vi "Path length, indv indice.vi"(11 "Raw position":dbl[][](array[numeric])) -> (3 "Path length data":dbl[][](array[numeric]))   [LabVIEW 2020]
panel:
  out "Path lenght data":dbl[](array[numeric])
  out "deleted portion":dbl[][](array[numeric])
  out "Path length upper shoulder":dbl
  out "path lenght Wrist":dbl
  out "path lenght elbow":dbl
  out "path lenght lower shoulder":dbl
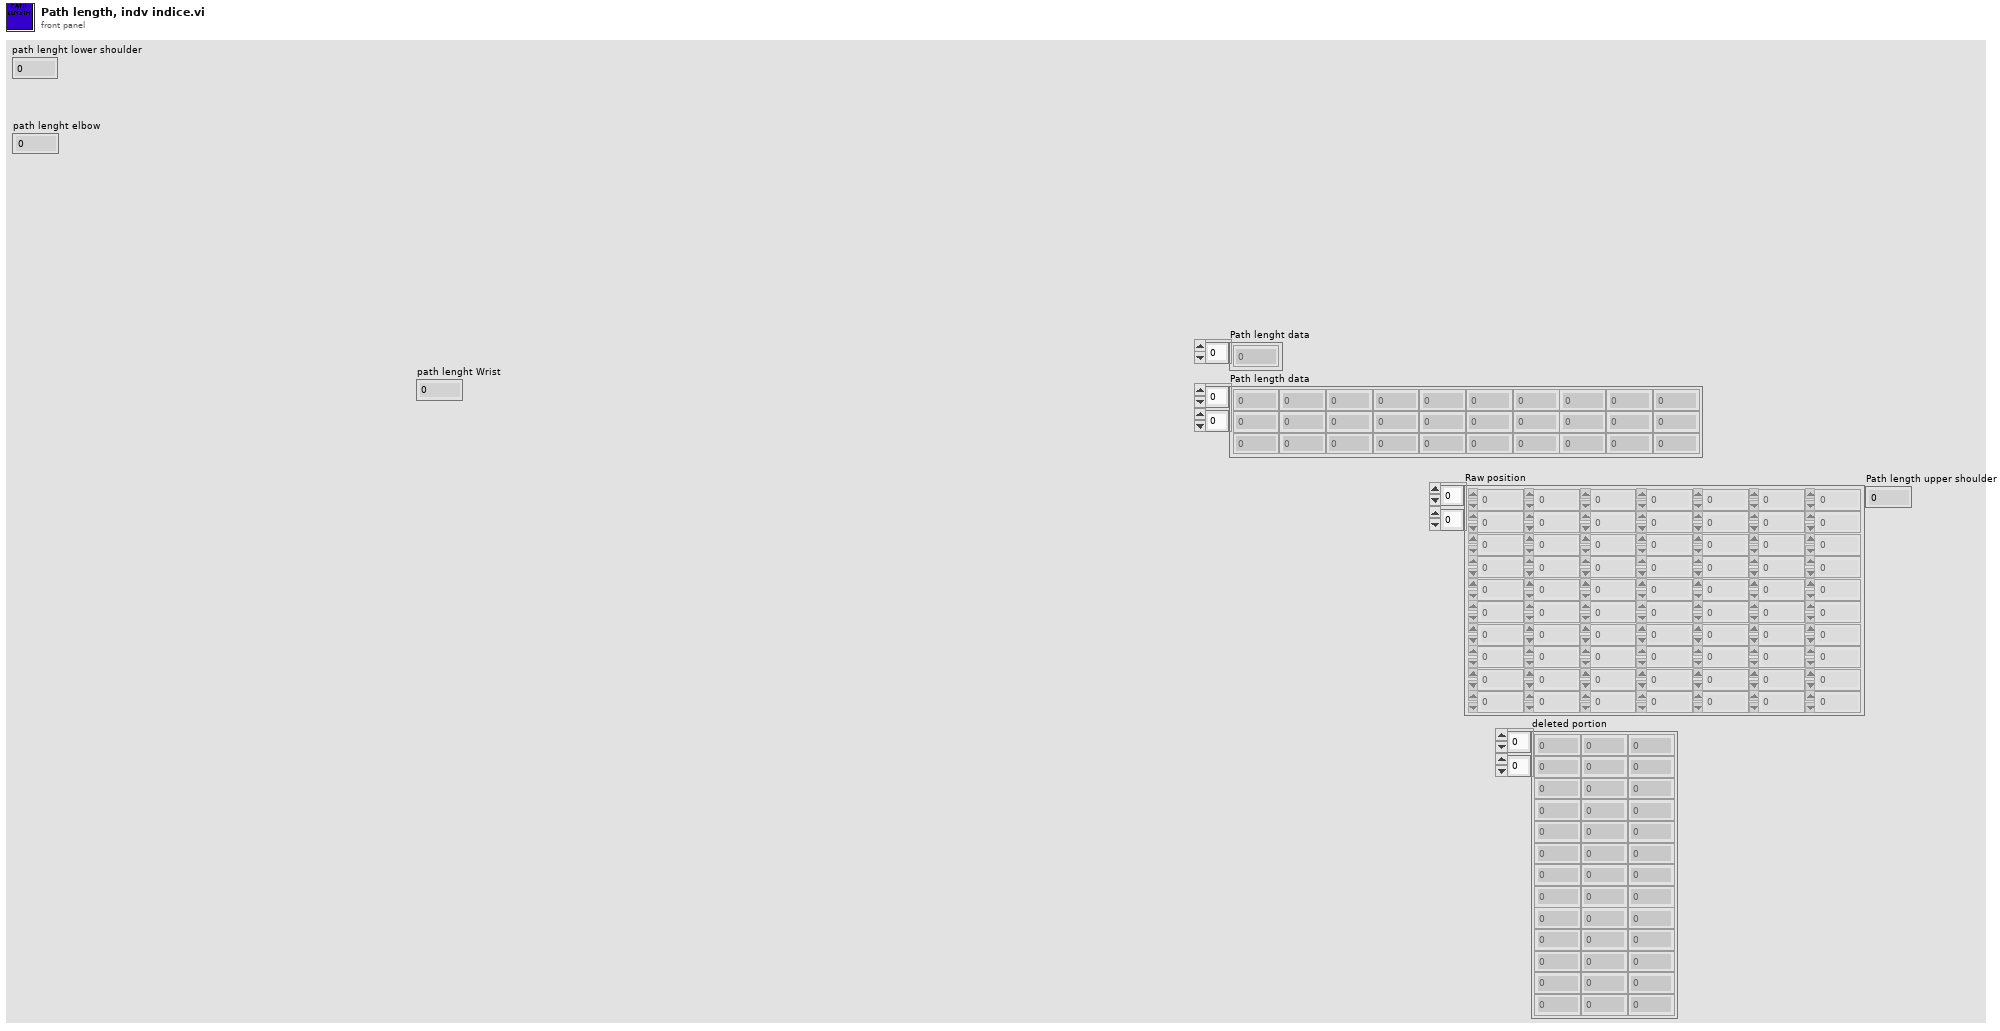
[diagram p1: front panel]
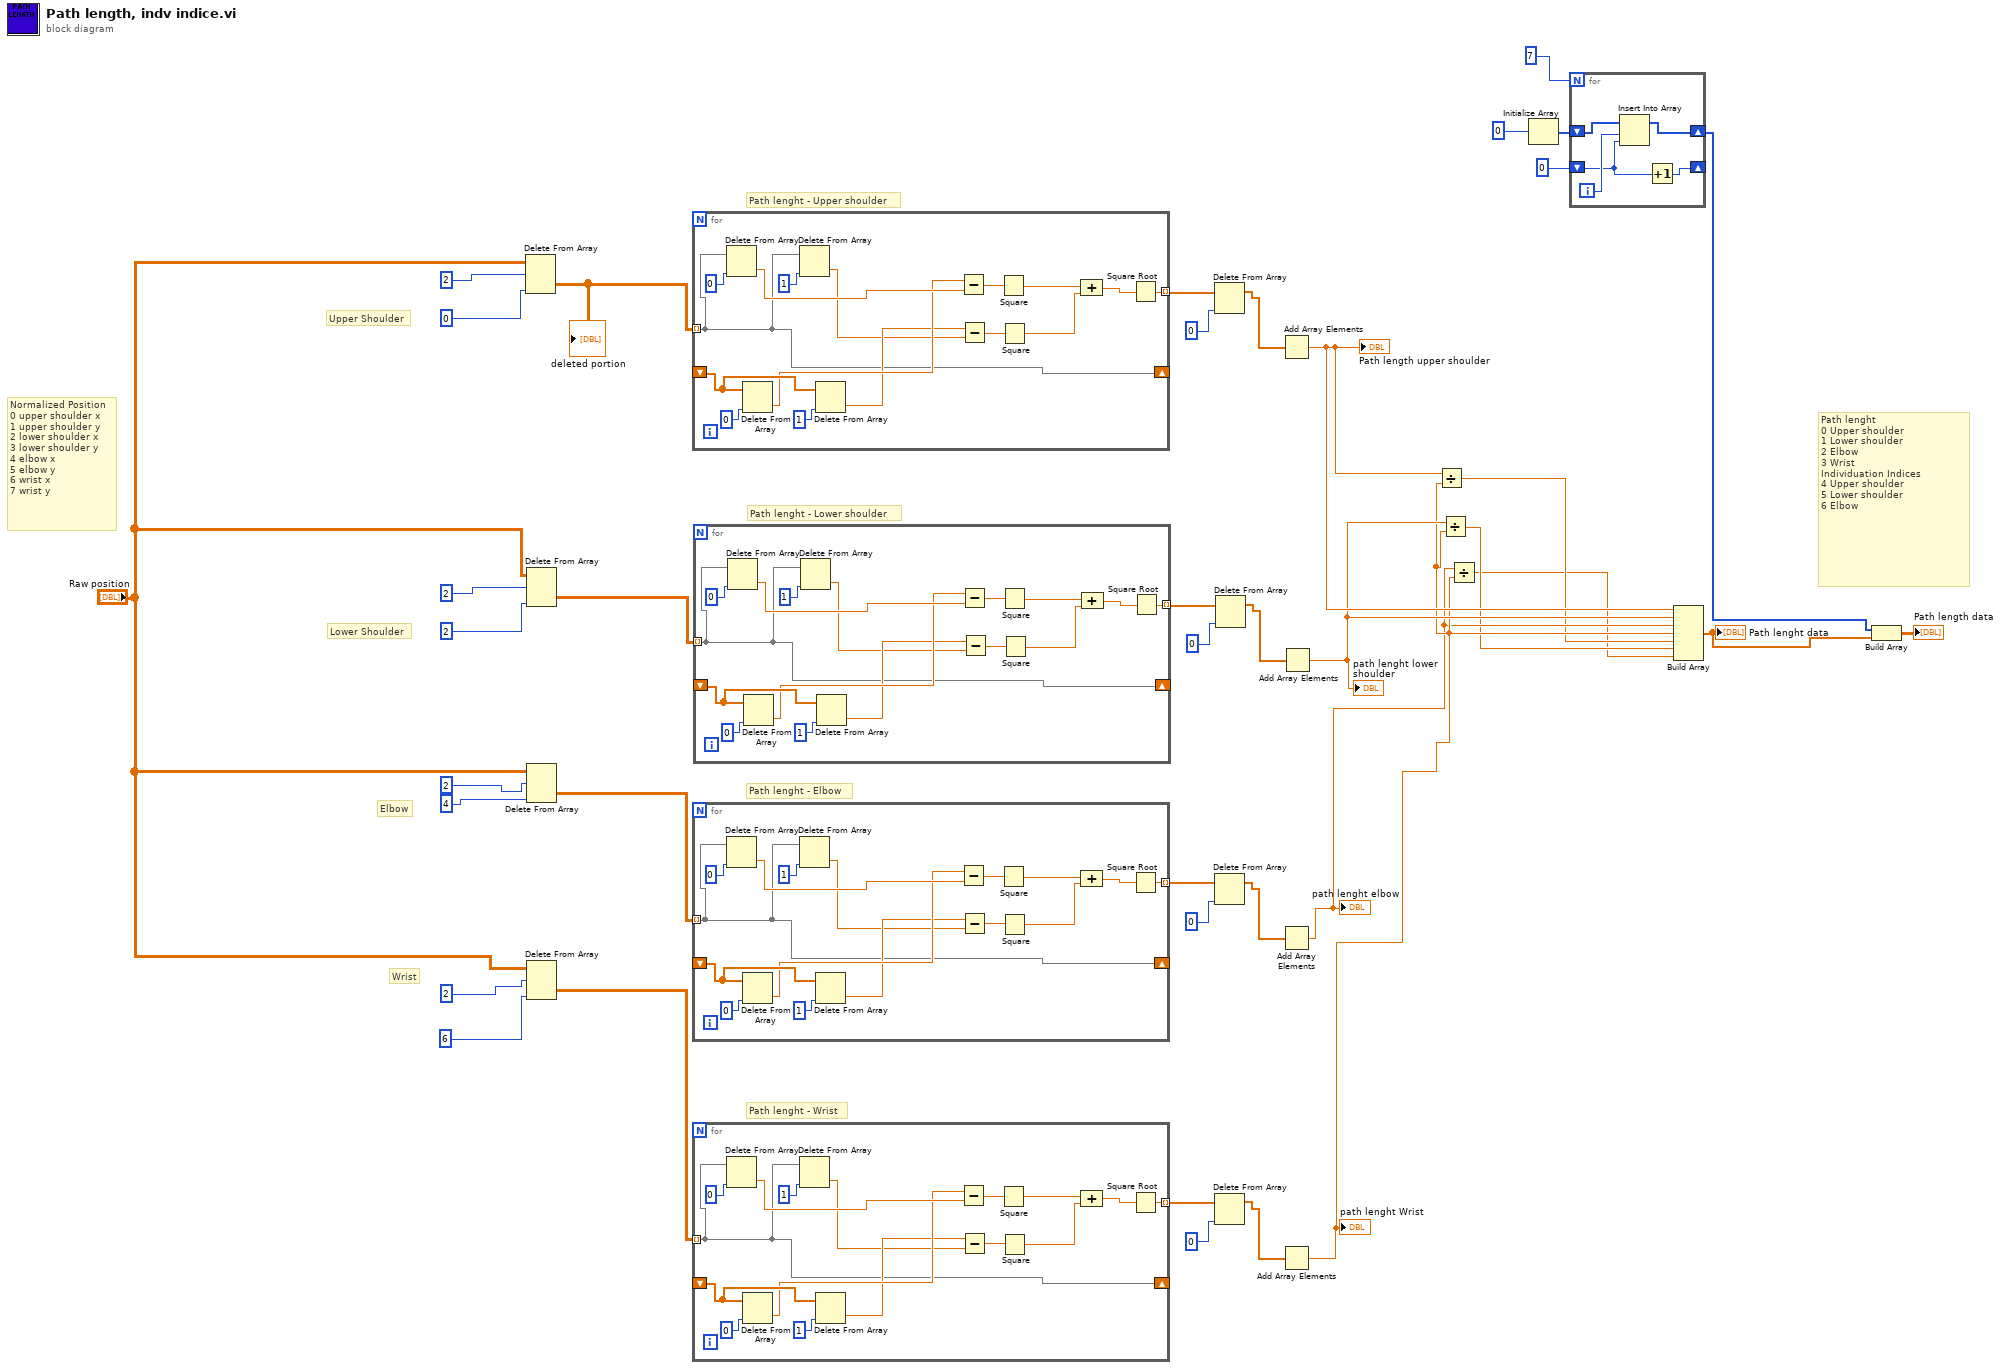
[diagram p0: block diagram]
diagram:
  # "Normalized Position\n0 upper shoulder x\n1 upper shoulder y\n2 lower shoulder x\n3 lower shoulder y\n4 elbow x\n5 elbow y\n6 wrist x\n7 wrist y"
  # "Path lenght - Upper shoulder"
  # "Upper Shoulder"
  # "Path lenght - Wrist"
  # "Path lenght - Elbow"
  # "Path lenght - Lower shoulder"
  # "Path lenght\n0 Upper shoulder\n1 Lower shoulder\n2 Elbow\n3 Wrist\nIndividuation Indices\n4 Upper shoulder\n5 Lower shoulder\n6 Elbow"
  # "Wrist"
  # "Elbow"
  # "Lower Shoulder"
  n1 = Delete From Array(array="Raw position", length=2, index (col)=0) -> (deleted portion=w17:dbl[][])  [unwired: 1 in, 1 out]
  "deleted portion" <- w17
  n2 = Delete From Array(array="Raw position", length=2, index (col)=2) -> (deleted portion=w33:dbl[][])  [unwired: 1 in, 1 out]
  n3 = Delete From Array(array="Raw position", length=2, index (col)=4) -> (deleted portion=w27:dbl[][])  [unwired: 1 in, 1 out]
  n4 = Delete From Array(array="Raw position", length=2, index (col)=6) -> (deleted portion=w22:dbl[][])  [unwired: 1 in, 1 out]
  n5 = for {
    shift-right: [w40] -> _
    shift-left: _ -> [w51]
    tunnel: w17 -> [w40] mode=indexing
    tunnel: [w41] -> w20 mode=indexing
    n6 = Delete From Array(array=w40, index=0) -> (deleted portion=w50:dbl)  [unwired: 1 in, 1 out]
    n7 = Delete From Array(array=w51, index=0) -> (deleted portion=w49:dbl)  [unwired: 1 in, 1 out]
    n8 = Delete From Array(array=w40, index=1) -> (deleted portion=w45:dbl)  [unwired: 1 in, 1 out]
    n9 = Delete From Array(array=w51, index=1) -> (deleted portion=w46:dbl)  [unwired: 1 in, 1 out]
    n10 = Subtract(x=w49, y=w50) -> (x-y=w48:dbl)
    n11 = Subtract(x=w46, y=w45) -> (x-y=w47:dbl)
    n12 = Square(x=w48) -> (x^2=w44:dbl)
    n13 = Square(x=w47) -> (x^2=w43:dbl)
    n14 = Compound Arithmetic op=ADD(w44, w43) -> (w42:dbl)
    n15 = Square Root(x=w42) -> (sqrt(x)=w41:dbl)
  }
  n16 = for {
    shift-right: [w56] -> _
    shift-left: _ -> [w67]
    tunnel: w27 -> [w56] mode=indexing
    tunnel: [w57] -> w31 mode=indexing
    n17 = Delete From Array(array=w56, index=0) -> (deleted portion=w66:dbl)  [unwired: 1 in, 1 out]
    n18 = Delete From Array(array=w67, index=0) -> (deleted portion=w65:dbl)  [unwired: 1 in, 1 out]
    n19 = Delete From Array(array=w56, index=1) -> (deleted portion=w61:dbl)  [unwired: 1 in, 1 out]
    n20 = Delete From Array(array=w67, index=1) -> (deleted portion=w62:dbl)  [unwired: 1 in, 1 out]
    n21 = Subtract(x=w65, y=w66) -> (x-y=w64:dbl)
    n22 = Subtract(x=w62, y=w61) -> (x-y=w63:dbl)
    n23 = Square(x=w64) -> (x^2=w60:dbl)
    n24 = Square(x=w63) -> (x^2=w59:dbl)
    n25 = Compound Arithmetic op=ADD(w60, w59) -> (w58:dbl)
    n26 = Square Root(x=w58) -> (sqrt(x)=w57:dbl)
  }
  n27 = for {
    shift-right: [w72] -> _
    shift-left: _ -> [w83]
    tunnel: w22 -> [w72] mode=indexing
    tunnel: [w73] -> w25 mode=indexing
    n28 = Delete From Array(array=w72, index=0) -> (deleted portion=w82:dbl)  [unwired: 1 in, 1 out]
    n29 = Delete From Array(array=w83, index=0) -> (deleted portion=w81:dbl)  [unwired: 1 in, 1 out]
    n30 = Delete From Array(array=w72, index=1) -> (deleted portion=w77:dbl)  [unwired: 1 in, 1 out]
    n31 = Delete From Array(array=w83, index=1) -> (deleted portion=w78:dbl)  [unwired: 1 in, 1 out]
    n32 = Subtract(x=w81, y=w82) -> (x-y=w80:dbl)
    n33 = Subtract(x=w78, y=w77) -> (x-y=w79:dbl)
    n34 = Square(x=w80) -> (x^2=w76:dbl)
    n35 = Square(x=w79) -> (x^2=w75:dbl)
    n36 = Compound Arithmetic op=ADD(w76, w75) -> (w74:dbl)
    n37 = Square Root(x=w74) -> (sqrt(x)=w73:dbl)
  }
  n38 = for {
    shift-right: [w88] -> _
    shift-left: _ -> [w99]
    tunnel: w33 -> [w88] mode=indexing
    tunnel: [w89] -> w36 mode=indexing
    n39 = Delete From Array(array=w88, index=0) -> (deleted portion=w98:dbl)  [unwired: 1 in, 1 out]
    n40 = Delete From Array(array=w99, index=0) -> (deleted portion=w97:dbl)  [unwired: 1 in, 1 out]
    n41 = Delete From Array(array=w88, index=1) -> (deleted portion=w93:dbl)  [unwired: 1 in, 1 out]
    n42 = Delete From Array(array=w99, index=1) -> (deleted portion=w94:dbl)  [unwired: 1 in, 1 out]
    n43 = Subtract(x=w97, y=w98) -> (x-y=w96:dbl)
    n44 = Subtract(x=w94, y=w93) -> (x-y=w95:dbl)
    n45 = Square(x=w96) -> (x^2=w92:dbl)
    n46 = Square(x=w95) -> (x^2=w91:dbl)
    n47 = Compound Arithmetic op=ADD(w92, w91) -> (w90:dbl)
    n48 = Square Root(x=w90) -> (sqrt(x)=w89:dbl)
  }
  n49 = Delete From Array(array=w20, index=0) -> (array with subset deleted=w18:dbl[])  [unwired: 1 in, 1 out]
  n50 = Delete From Array(array=w31, index=0) -> (array with subset deleted=w29:dbl[])  [unwired: 1 in, 1 out]
  n51 = Delete From Array(array=w25, index=0) -> (array with subset deleted=w23:dbl[])  [unwired: 1 in, 1 out]
  n52 = Delete From Array(array=w36, index=0) -> (array with subset deleted=w34:dbl[])  [unwired: 1 in, 1 out]
  n53 = Add Array Elements(numeric array=w18) -> (sum=w10:dbl)
  "Path length upper shoulder" <- w10
  n54 = Add Array Elements(numeric array=w29) -> (sum=w7:dbl)
  "path lenght elbow" <- w7
  n55 = Add Array Elements(numeric array=w23) -> (sum=w8:dbl)
  "path lenght Wrist" <- w8
  n56 = Add Array Elements(numeric array=w34) -> (sum=w9:dbl)
  "path lenght lower shoulder" <- w9
  n57 = Divide(x=w10, y=w8) -> (x/y=w6:dbl)
  n58 = Divide(x=w9, y=w8) -> (x/y=w5:dbl)
  n59 = Divide(x=w7, y=w8) -> (x/y=w4:dbl)
  n60 = Initialize Array(0) -> (w12:i32[])  [unwired: 1 in]
  n61 = for {
    N: 7 -> [_]
    shift-right: [w106] -> w3
    shift-left: w12 -> [w107]
    shift-right: [w104] -> _
    shift-left: 0 -> [w105]
    i -> [w108]
    n62 = Insert Into Array(array=w107, index=w108, new element=w105) -> (w106:i32[])
    n63 = Increment(x=w105) -> (x+1=w104:i32)
  }
  n64 = Build Array(w10, w9, w7, w8, w6, w5, w4) -> (w2:dbl[])
  "Path lenght data" <- w2
  n65 = Build Array(w3, w2) -> (→"Path length data":dbl[][])
